vi "CDIR To Byte.vi"(11 "DIR":T1) -> (3 "Numeric":u8)   [LabVIEW 2022 SP3, in "FHPP.lvclass"]
uses:
  FHPP.lvclass
  FHPP.lvclass/FHPP.ctl
  DIR.ctl
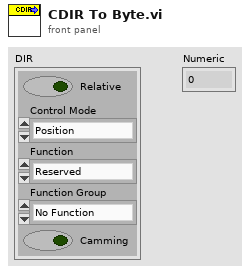
[diagram p1: front panel]
types:
  T1 = typedef "FHPP.lvclass/DIR.ctl" = cluster{"Relative":bool, "Control Mode":enum8{"Position", "Force", "Velocity", "Reserved"}, "Function":enum8{"Reserved", "External Input", "External Input with  Cam", "Virtual Master with Cam"}, "Function Group":enum8{"No Function", "Reserver 1", "Reserved 2", "Reserved 3"}, "Camming":bool}
  T2 = enum8{"Position", "Force", "Velocity", "Reserved"}
  T3 = enum8{"Reserved", "External Input", "External Input with  Cam", "Virtual Master with Cam"}
  T4 = enum8{"No Function", "Reserver 1", "Reserved 2", "Reserved 3"}
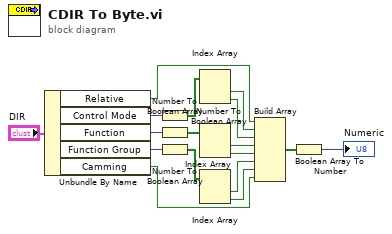
[diagram p0: block diagram]
diagram:
  n1 = Unbundle By Name("DIR") -> ("Relative"=w8:bool, "Control Mode"=w2:T2, "Function"=w3:T3, "Function Group"=w4:T4, "Camming"=w15:bool)
  n2 = Number To Boolean Array(number=w2) -> (Boolean array=w5:bool[])
  n3 = Number To Boolean Array(number=w3) -> (Boolean array=w6:bool[])
  n4 = Number To Boolean Array(number=w4) -> (Boolean array=w7:bool[])
  n5 = Index Array(array=w5) -> (element #1=w9:bool, element #2=w10:bool)  [unwired: 2 in]
  n6 = Index Array(array=w6) -> (element #1=w11:bool, element #2=w12:bool)  [unwired: 2 in]
  n7 = Index Array(array=w7) -> (element #1=w13:bool, element #2=w14:bool)  [unwired: 2 in]
  n8 = Build Array(w8, w9, w10, w11, w12, w13, w14, w15) -> (w16:bool[])
  n9 = Boolean Array To Number(Boolean array=w16) -> (number=→"Numeric":u8)
